vi "LogError.vi"(8 "error in (no error)":errorcluster, 9 "error":errorcluster, 11 "qbus in":refnum<class "Qbus.lvclass">) -> (0 "error out":errorcluster, 3 "qbus out":refnum<class "Qbus.lvclass">)   [LabVIEW 2017, in "TraceLogger.lvlib"]
doc: "Logs a tracepoint instance that includes the error code and the source of an error within an error cluster. To specify a custom error string rather than the source, use the Log Error String VI instead."
uses:
  <vilib>/addons/TraceLogger/TraceLogger.lvlib
  <vilib>/addons/Qbus/Qbus.lvclass
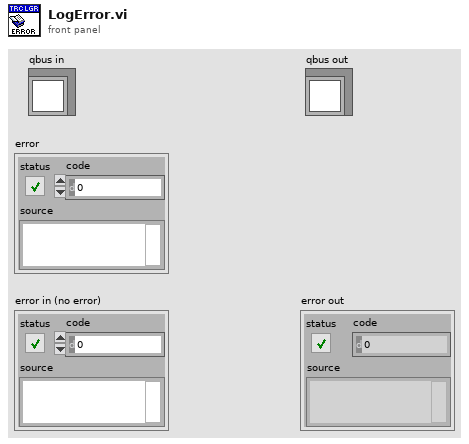
[diagram p1: front panel]
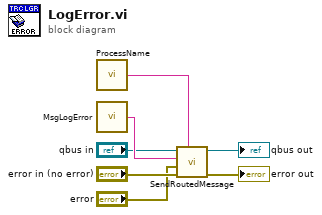
[diagram p0: block diagram]
diagram:
  n1 = call <vilib>:"ProcessName.vi"() -> ("process name"=w4:string)  [unwired: 5 in]
  n2 = call <vilib>:"MsgLogError.vi"() -> ("message name"=w6:string)  [unwired: 5 in]
  n3 = call <vilib>:"SendRoutedMessage.vi"("listener process"=w4, "error in (no error)"="error in (no error)", "message value"="error", "message name"=w6, "Qbus in"="qbus in") -> ("error in (no error)"=→"error out":errorcluster, "Qbus out"=→"qbus out":refnum<class "Qbus.lvclass">)  [unwired: 5 in]
